vi "GetEventAppliedAberrationForcesField.vi"(10 "Event Data":string, 11 "Cluster in":refnum<vi>) -> (3 "Array":string[](array[string]))   [LabVIEW 2016]
uses:
  SALLV_m1m3/DataTypes/logevent_AppliedAberrationForces.ctl
  SALLV_m1m3/SALLV_m1m3.lvlib
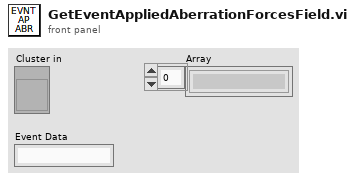
[diagram p1: front panel]
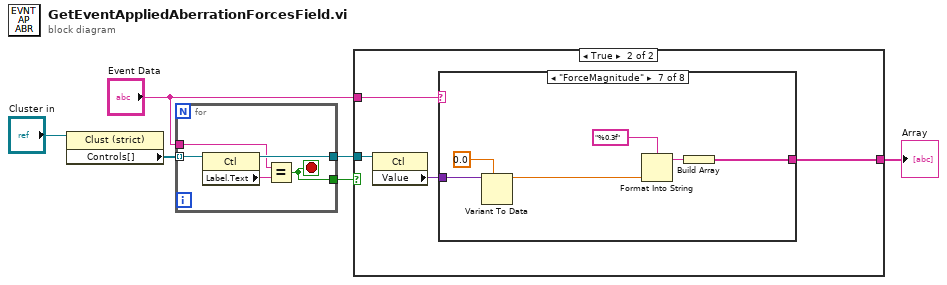
[diagram p0: block diagram]
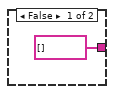
[diagram p2: hidden frame]
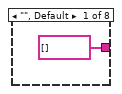
[diagram p3: hidden frame]
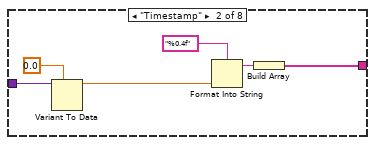
[diagram p4: hidden frame]
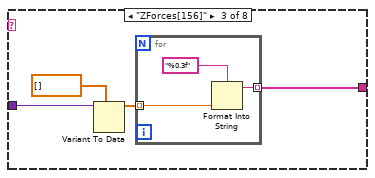
[diagram p5: hidden frame]
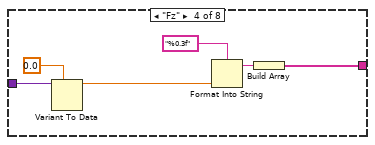
[diagram p6: hidden frame]
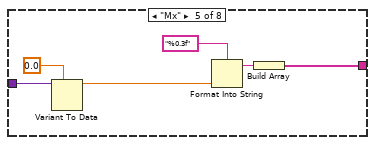
[diagram p7: hidden frame]
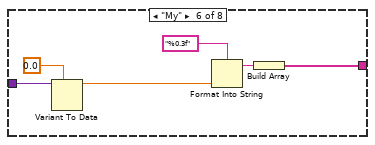
[diagram p8: hidden frame]
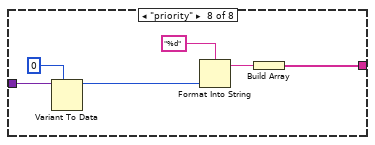
[diagram p9: hidden frame]
diagram:
  n1 = property on="Property Node" class="Clust (strict)"(reference="Cluster in") -> ("Controls[]"=w6:refnum<vi>[])  [unwired: 1 in, 2 out]
  n2 = for {
    tunnel: w6 -> [w11] mode=indexing
    tunnel: [w10] -> w4
    tunnel: "Event Data" -> [w8]
    tunnel: [w7] -> w5
    stop <- w7 stop-if-true
    n3 = property on="Property Node" class="Ctl"(reference=w11) -> (reference out=w10:refnum<vi>, "Label.Text"=w9:string)  [unwired: 1 in, 1 out]
    n4 = Equal?(x=w8, y=w9) -> (x = y?=w7:bool)
  }
  n5 = case shown="True" w5 {
    tunnel: "Event Data" -> [_ w16]
    tunnel: w4 -> [_ w15]
    tunnel: [string[] [] w13] -> w2
    frame False {
    }
    frame True {
      n6 = property on="Property Node" class="Ctl"(reference=w15) -> ("Value"=w14:variant)  [unwired: 1 in, 2 out]
      n7 = case shown="\"ForceMagnitude\"" w16 {
        tunnel: [string[] [] w21 w24 w34 w40 w46 w52 w58] -> w13
        tunnel: w14 -> [_ w19 w27 w32 w38 w44 w50 w56]
        frame "", Default {
        }
        frame "Timestamp" {
          n8 = Variant To Data(type=0.0, Variant=w19) -> (data=w20:dbl)  [unwired: 1 in, 1 out]
          n9 = Format Into String(format string="%0.4f", w20) -> (resulting string=w22:string)  [unwired: 2 in, 1 out]
          n10 = Build Array(w22) -> (w21:string[])
        }
        frame "ZForces[156]" {
          n11 = Variant To Data(type=sgl[] [], Variant=w27) -> (data=w25:sgl[])  [unwired: 1 in, 1 out]
          n12 = for {
            tunnel: w25 -> [w29] mode=indexing
            tunnel: [w28] -> w24 mode=indexing
            n13 = Format Into String(format string="%0.3f", w29) -> (resulting string=w28:string)  [unwired: 2 in, 1 out]
          }
        }
        frame "Fz" {
          n14 = Variant To Data(type=0.0, Variant=w32) -> (data=w33:dbl)  [unwired: 1 in, 1 out]
          n15 = Format Into String(format string="%0.3f", w33) -> (resulting string=w35:string)  [unwired: 2 in, 1 out]
          n16 = Build Array(w35) -> (w34:string[])
        }
        frame "Mx" {
          n17 = Variant To Data(type=0.0, Variant=w38) -> (data=w39:dbl)  [unwired: 1 in, 1 out]
          n18 = Format Into String(format string="%0.3f", w39) -> (resulting string=w41:string)  [unwired: 2 in, 1 out]
          n19 = Build Array(w41) -> (w40:string[])
        }
        frame "My" {
          n20 = Variant To Data(type=0.0, Variant=w44) -> (data=w45:dbl)  [unwired: 1 in, 1 out]
          n21 = Format Into String(format string="%0.3f", w45) -> (resulting string=w47:string)  [unwired: 2 in, 1 out]
          n22 = Build Array(w47) -> (w46:string[])
        }
        frame "ForceMagnitude" {
          n23 = Variant To Data(type=0.0, Variant=w50) -> (data=w51:dbl)  [unwired: 1 in, 1 out]
          n24 = Format Into String(format string="%0.3f", w51) -> (resulting string=w53:string)  [unwired: 2 in, 1 out]
          n25 = Build Array(w53) -> (w52:string[])
        }
        frame "priority" {
          n26 = Variant To Data(type=0, Variant=w56) -> (data=w57:i32)  [unwired: 1 in, 1 out]
          n27 = Format Into String(format string="%d", w57) -> (resulting string=w59:string)  [unwired: 2 in, 1 out]
          n28 = Build Array(w59) -> (w58:string[])
        }
      }
    }
  }
  "Array" <- w2
